vi "SCMP - picture flip rotate.vi"(8 "D":u32[][](array[numeric]), 9 "C":u32[][](array[numeric]), 10 "B":u32[][](array[numeric]), 11 "A":u32[][](array[numeric])) -> (0 "Array D":u32[][](array[numeric]), 1 "Array C":u32[][](array[numeric]), 2 "Array B":u32[][](array[numeric]), 3 "Array A":u32[][](array[numeric]))   [LabVIEW 2014]
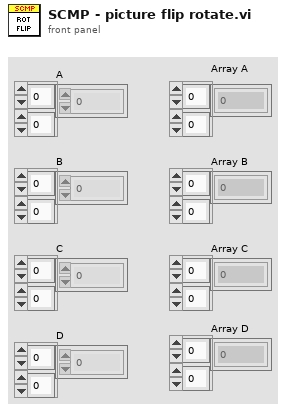
[diagram p1: front panel]
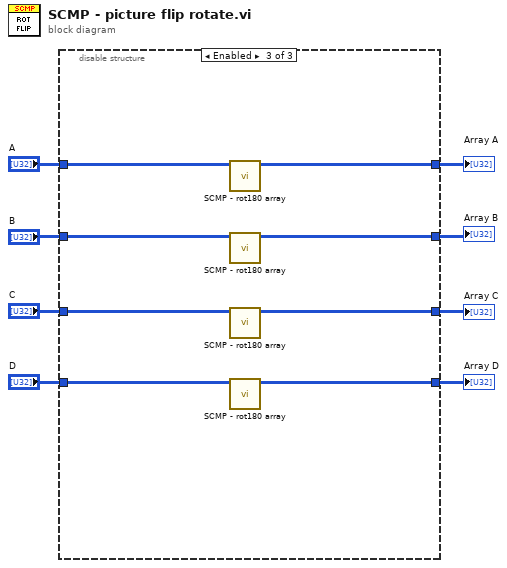
[diagram p0: block diagram]
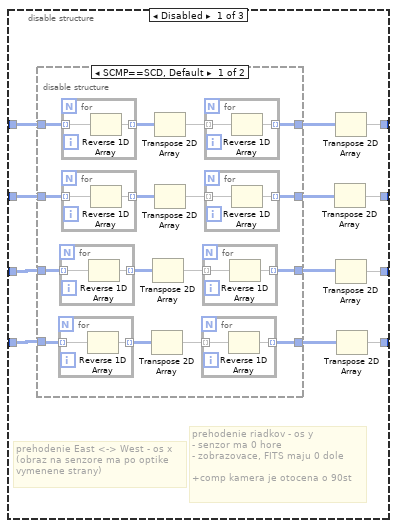
[diagram p2: hidden frame]
diagram:
  n1 = disable-structure shown="Enabled" {
    disable-tunnel: [w19 w59 w65] -> w8
    disable-tunnel: "B" -> [w16 w59 w66]
    disable-tunnel: "A" -> [w15 w60 w68]
    disable-tunnel: [w14 w57 w61] -> w5
    disable-tunnel: "D" -> [w13 w57 w62]
    disable-tunnel: [w11 w60 w67] -> w3
    disable-tunnel: "C" -> [w10 w58 w64]
    disable-tunnel: [w9 w58 w63] -> w1
    frame Disabled {
      # "prehodenie East <-> West - os x\n(obraz na senzore ma po optike \nvymenene strany)"
      # "prehodenie riadkov - os y\n- senzor ma 0 hore\n- zobrazovace, FITS maju 0 dole\n\n+comp kamera je otocena o 90st"
      n2 = disable-structure shown="SCMP==SCD, Default" {
        disable-tunnel: w13 -> [w36 w56]
        disable-tunnel: [w33 w56] -> w12
        disable-tunnel: w15 -> [w26 w53]
        disable-tunnel: w16 -> [w25 w54]
        disable-tunnel: w10 -> [w24 w55]
        disable-tunnel: [w23 w55] -> w17
        disable-tunnel: [w22 w54] -> w18
        disable-tunnel: [w21 w53] -> w20
        frame condition #0 {
          n3 = for {
            tunnel: w36 -> [w52] mode=indexing
            tunnel: [w51] -> w35 mode=indexing
            n4 = Reverse 1D Array(array=w52) -> (reversed array=w51:u32[])
          }
          n5 = for {
            tunnel: w24 -> [w48] mode=indexing
            tunnel: [w47] -> w32 mode=indexing
            n6 = Reverse 1D Array(array=w48) -> (reversed array=w47:u32[])
          }
          n7 = for {
            tunnel: w26 -> [w40] mode=indexing
            tunnel: [w39] -> w28 mode=indexing
            n8 = Reverse 1D Array(array=w40) -> (reversed array=w39:u32[])
          }
          n9 = for {
            tunnel: w25 -> [w44] mode=indexing
            tunnel: [w43] -> w30 mode=indexing
            n10 = Reverse 1D Array(array=w44) -> (reversed array=w43:u32[])
          }
          n11 = Transpose 2D Array(2D array=w35) -> (transposed array=w34:u32[][])
          n12 = Transpose 2D Array(2D array=w32) -> (transposed array=w31:u32[][])
          n13 = Transpose 2D Array(2D array=w28) -> (transposed array=w27:u32[][])
          n14 = Transpose 2D Array(2D array=w30) -> (transposed array=w29:u32[][])
          n15 = for {
            tunnel: w34 -> [w50] mode=indexing
            tunnel: [w49] -> w33 mode=indexing
            n16 = Reverse 1D Array(array=w50) -> (reversed array=w49:u32[])
          }
          n17 = for {
            tunnel: w31 -> [w46] mode=indexing
            tunnel: [w45] -> w23 mode=indexing
            n18 = Reverse 1D Array(array=w46) -> (reversed array=w45:u32[])
          }
          n19 = for {
            tunnel: w27 -> [w38] mode=indexing
            tunnel: [w37] -> w21 mode=indexing
            n20 = Reverse 1D Array(array=w38) -> (reversed array=w37:u32[])
          }
          n21 = for {
            tunnel: w29 -> [w42] mode=indexing
            tunnel: [w41] -> w22 mode=indexing
            n22 = Reverse 1D Array(array=w42) -> (reversed array=w41:u32[])
          }
        }
        frame condition #1 (active) {
        }
      }
      n23 = Transpose 2D Array(2D array=w18) -> (transposed array=w19:u32[][])
      n24 = Transpose 2D Array(2D array=w20) -> (transposed array=w11:u32[][])
      n25 = Transpose 2D Array(2D array=w17) -> (transposed array=w9:u32[][])
      n26 = Transpose 2D Array(2D array=w12) -> (transposed array=w14:u32[][])
    }
    frame Disabled {
    }
    frame Enabled {
      n27 = call "SCMP - rot180 array.vi"("A in"=w68) -> ("A out"=w67:u32[][])  [unwired: 10 in]
      n28 = call "SCMP - rot180 array.vi"("A in"=w66) -> ("A out"=w65:u32[][])  [unwired: 10 in]
      n29 = call "SCMP - rot180 array.vi"("A in"=w64) -> ("A out"=w63:u32[][])  [unwired: 10 in]
      n30 = call "SCMP - rot180 array.vi"("A in"=w62) -> ("A out"=w61:u32[][])  [unwired: 10 in]
    }
  }
  "Array B" <- w8
  "Array C" <- w1
  "Array D" <- w5
  "Array A" <- w3
